vi "RT1.vi"(6 "ErrorIn":errorcluster, 8 "InCluster":T3, 9 "Reference":T1) -> (0 "ErrorOut":errorcluster, 2 "OutCluster":T2, 3 "ReferenceOut":T1)   [LabVIEW 2022 SP3]
uses:
  C:/Users/Robots/Documents/robocadSimLV/assemblies/LibraryForLabVIEW.dll
  assemblies/LibraryForLabVIEW.dll
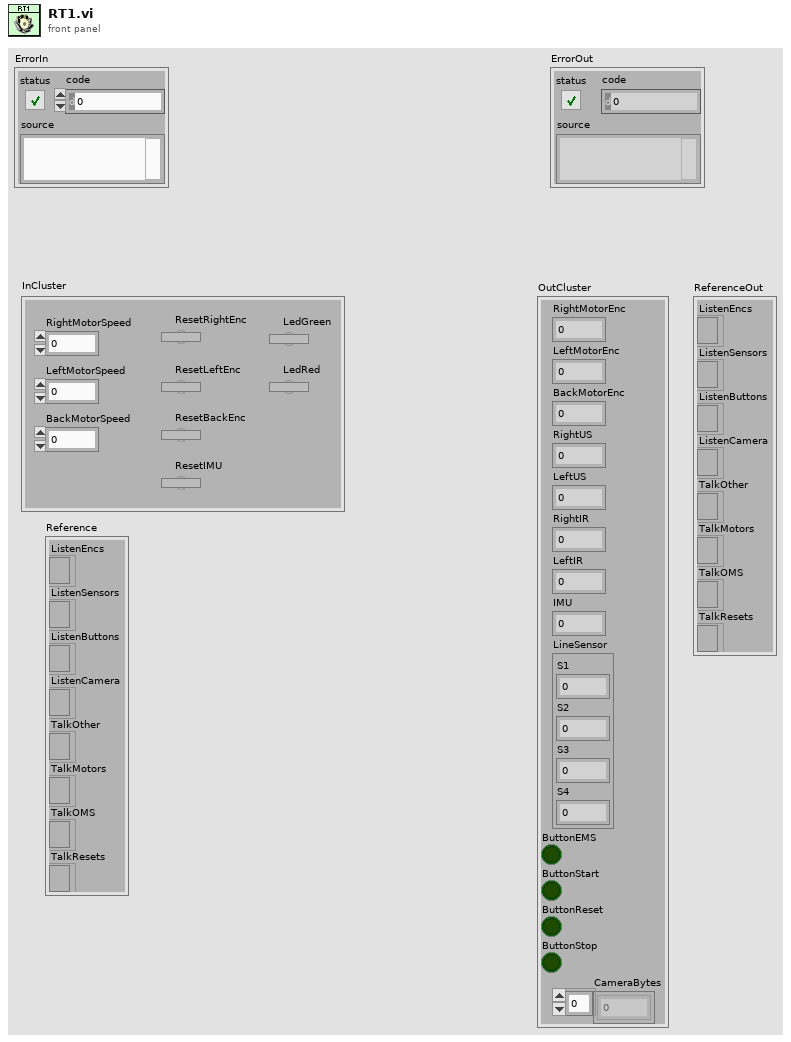
[diagram p1: front panel]
types:
  T1 = cluster{"ListenEncs":refnum<k24>, "ListenSensors":refnum<k24>, "ListenButtons":refnum<k24>, "ListenCamera":refnum<k24>, "TalkOther":refnum<k24>, "TalkMotors":refnum<k24>, "TalkOMS":refnum<k24>, "TalkResets":refnum<k24>}
  T2 = cluster{"RightMotorEnc":dbl, "LeftMotorEnc":dbl, "BackMotorEnc":dbl, "RightUS":dbl, "LeftUS":dbl, "RightIR":dbl, "LeftIR":dbl, "IMU":dbl, "LineSensor":cluster{"S1":dbl, "S2":dbl, "S3":dbl, "S4":dbl}, "ButtonEMS":bool, "ButtonStart":bool, "ButtonReset":bool, "ButtonStop":bool, "CameraBytes":u8[]}
  T3 = cluster{"RightMotorSpeed":dbl, "LeftMotorSpeed":dbl, "BackMotorSpeed":dbl, "ResetRightEnc":bool, "ResetLeftEnc":bool, "ResetBackEnc":bool, "ResetIMU":bool, "LedGreen":bool, "LedRed":bool}
  T4 = cluster{"Encs":dbl[], "Sensors":dbl[], "Buttons":bool[], "Camera":u8[]}
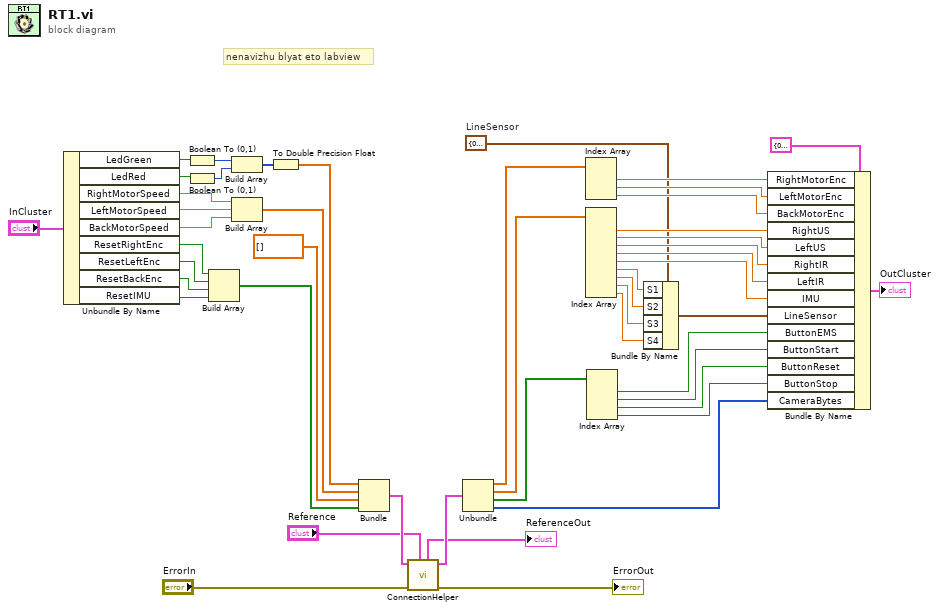
[diagram p0: block diagram]
diagram:
  w15 = cluster{"S1":dbl, "S2":dbl, "S3":dbl, "S4":dbl} {"S1"=0.0, "S2"=0.0, "S3"=0.0, "S4"=0.0}  # LineSensor
  # "nenavizhu blyat eto labview"
  n1 = Unbundle By Name("InCluster") -> ("LedGreen"=w40:bool, "LedRed"=w39:bool, "RightMotorSpeed"=w43:dbl, "LeftMotorSpeed"=w44:dbl, "BackMotorSpeed"=w42:dbl, "ResetRightEnc"=w32:bool, "ResetLeftEnc"=w33:bool, "ResetBackEnc"=w34:bool, "ResetIMU"=w35:bool)
  n2 = Boolean To (0,1)(Boolean=w40) -> (0, 1=w38:i16)
  n3 = Boolean To (0,1)(Boolean=w39) -> (0, 1=w37:i16)
  n4 = Build Array(w32, w33, w34, w35) -> (w31:bool[])
  n5 = Build Array(w38, w37) -> (w29:i16[])
  n6 = Build Array(w43, w44, w42) -> (w41:dbl[])
  n7 = To Double Precision Float(number=w29) -> (double precision float=w28:dbl[])
  n8 = Bundle(w28, w41, dbl[] [], w31) -> (w30:cluster{dbl[], dbl[], dbl[], bool[]})  [unwired: 1 in]
  n9 = call "ConnectionHelper.vi"("Reference"="Reference", "ErrorIn"="ErrorIn", "InCluster"=w30) -> ("ErrorOut"=→"ErrorOut":errorcluster, "OutCluster"=w27:T4, "ReferenceOut"=→"ReferenceOut":T1)  [unwired: 6 in]
  n10 = Unbundle(w27) -> ("Encs"=w26:dbl[], "Sensors"=w21:dbl[], "Buttons"=w9:bool[], "Camera"=w5:u8[])
  n11 = Index Array(array=w26) -> (element #1=w24:dbl, element #2=w23:dbl, element #3=w22:dbl)  [unwired: 3 in]
  n12 = Index Array(array=w21) -> (element #1=w20:dbl, element #2=w19:dbl, element #3=w18:dbl, element #4=w17:dbl, element #5=w16:dbl, element #6=w13:dbl, element #7=w12:dbl, element #8=w11:dbl, element #9=w10:dbl)  [unwired: 9 in]
  n13 = Index Array(array=w9) -> (element #1=w8:bool, element #2=w7:bool, element #3=w6:bool, element #4=w3:bool)  [unwired: 4 in]
  n14 = Bundle By Name(cluster=w15, "S1"=w13, "S2"=w12, "S3"=w11, "S4"=w10) -> (w14:cluster{"S1":dbl, "S2":dbl, "S3":dbl, "S4":dbl})
  n15 = Bundle By Name(cluster=T2 {"RightMotorEnc"=0.0, "LeftMotorEnc"=0.0, "BackMotorEnc"=0.0, "RightUS"=0.0, "LeftUS"=0.0, "RightIR"=0.0, "LeftIR"=0.0, "IMU"=0.0, "LineSensor"={"S1"=0.0, "S2"=0.0, "S3"=0.0, "S4"=0.0}, "ButtonEMS"=FALSE, "ButtonStart"=FALSE, "ButtonReset"=FALSE, "ButtonStop"=FALSE, "CameraBytes"=[]} ("input cluster"), "RightMotorEnc"=w24, "LeftMotorEnc"=w23, "BackMotorEnc"=w22, "RightUS"=w20, "LeftUS"=w19, "RightIR"=w18, "LeftIR"=w17, "IMU"=w16, "LineSensor"=w14, "ButtonEMS"=w8, "ButtonStart"=w7, "ButtonReset"=w6, "ButtonStop"=w3, "CameraBytes"=w5) -> (→"OutCluster":T2)
